vi "minExampleReadDataPackage.vi"() -> ()   [LabVIEW 2021]
panel:
  in  "length":i32
  out "Waveform Graph":dbl[][](graph)
  in  "Channels":i32=6
  in  "stop":bool
  in  "time readout loops [ms]":u32=500
  out "error in (no error)":errorcluster
  out "Error String Out":string
  in  "Boolean":bool
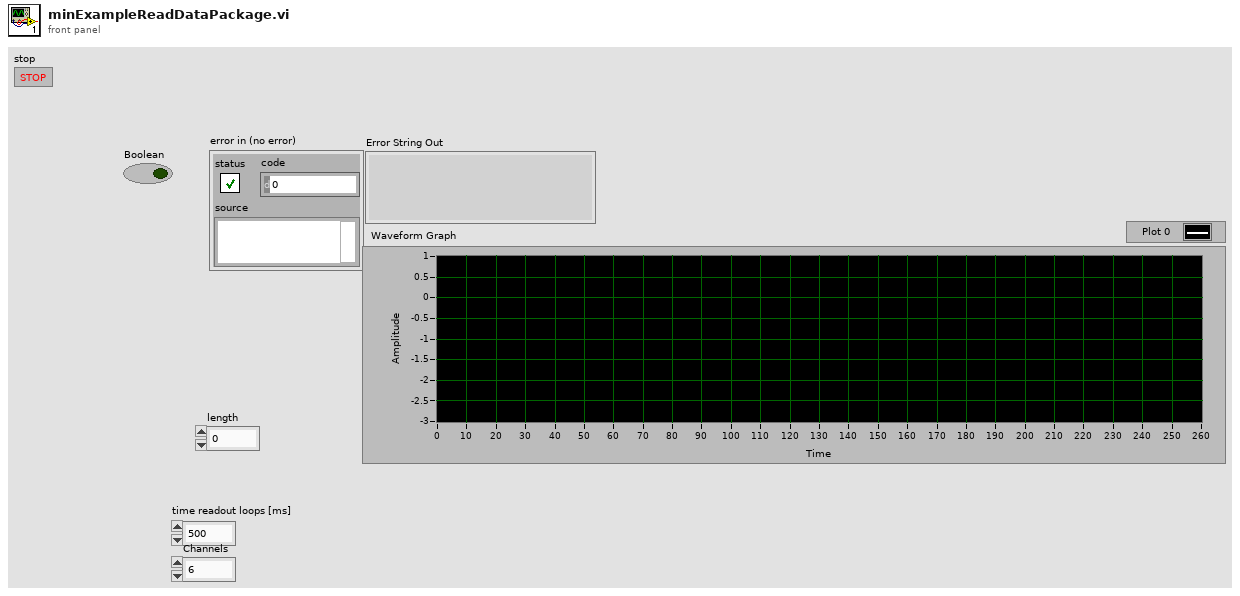
[diagram p1: front panel]
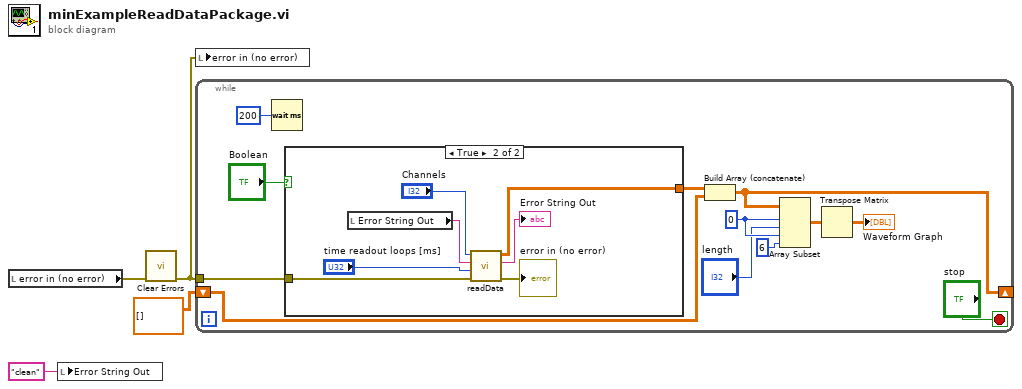
[diagram p0: block diagram]
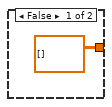
[diagram p2: hidden frame]
diagram:
  n1 = local read "error in (no error)"() -> (w4:errorcluster)
  n2 = local write "Error String Out"("clean" ("Error String Out")) -> ()
  n3 = call <vilib>:"Clear Errors.vi"("error in (no error)"=w4) -> ("error out"=w3:errorcluster)  [unwired: 5 in, 1 out]
  n4 = local write "error in (no error)"(w3) -> ()
  n5 = while {
    tunnel: w3 -> [w13]
    shift-right: [w7] -> _
    shift-left: dbl[][] [] -> [w11]
    stop <- "stop" stop-if-true
    w10 = 0 ("index")
    n6 = Wait (ms)(milliseconds to wait=u32 200) -> ()  [unwired: 1 out]
    n7 = case shown="True" "Boolean" {
      tunnel: w13 -> [_ w24]
      tunnel: [dbl[][] [] ("Array") w22] -> w12
      frame False {
      }
      frame True {
        n8 = local read "Error String Out"() -> (w18:string)
        n9 = call "readData.vi"("error in (no error)"=w24, "time readout loops [ms]"="time readout loops [ms]", "Error String Out in"=w18, "Channels"="Channels") -> ("error out"=→"error in (no error)":errorcluster, "Error String Out out"=→"Error String Out":string, "Array"=w22:dbl[][])  [unwired: 5 in]
      }
    }
    n10 = Build Array (concatenate)(w12, w11) -> (w7:dbl[][])
    n11 = Array Subset(array=w7, index (row)=w10, length (row)="length", index (col)=w10, length (col)=6 ("index (row)")) -> (w6:dbl[][])
    n12 = Transpose Matrix(1:w6) -> (0:→"Waveform Graph":dbl[][])
  }
